vi "Read configuration.vi"(7 "force loading?":bool=TRUE, 8 "error in (no error)":errorcluster, 11 "AOTF in":refnum<class "AOTF.lvclass">) -> (0 "error out":errorcluster, 3 "AOTF out":refnum<class "AOTF.lvclass">)   [LabVIEW 2012, in "AOTF.lvclass"]
doc: "Reads the XML-based configuration file and populates the configuration cluster accordingly. Configuration file name is <component ID>.xml."
uses:
  AOTF.lvclass
  <vilib>/Distrio/Murmex/Murmex/Murmex.lvclass
  AOTF.lvclass/AOTF.ctl
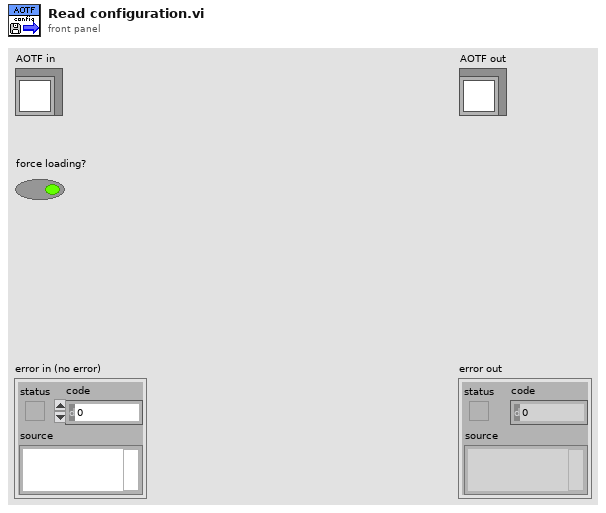
[diagram p1: front panel]
types:
  T1 = typedef "AOTF.lvclass/Configuration cluster.ctl" = cluster{"AO channel":string, "DO lines":string, "LUT path Cluster":cluster{"LUT path Array":path[]}}
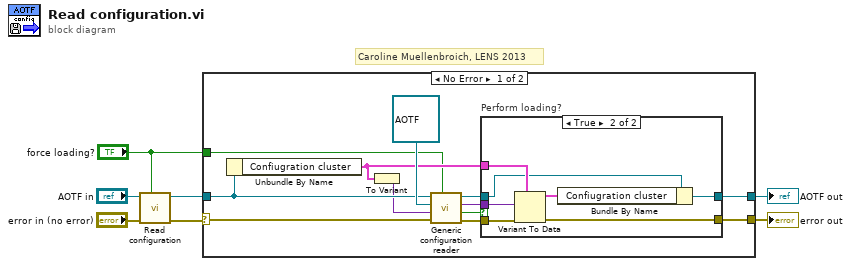
[diagram p0: block diagram]
diagram:
  # "Caroline Muellenbroich, LENS 2013"
  n1 = call-parent "Read configuration.vi"("force loading?"="force loading?", "error in (no error)"="error in (no error)", "Murmex in"="AOTF in") -> ("error out"=w5:errorcluster, "Murmex out"=w4:refnum<class "AOTF.lvclass">)  [unwired: 7 in]
  n2 = case shown="No Error" w5 {
    selector: w5 -> [w16 w30]
    tunnel: w4 -> [w14 w29]
    tunnel: [w18 w30] -> w3
    tunnel: [w19 w29] -> w2
    tunnel: "force loading?" -> [w11 _]
    frame No Error {
      n3 = Unbundle By Name(w14) -> ("Confiugration cluster"=w13:T1)
      n4 = To Variant(anything=w13) -> (Variant=w12:variant)
      n5 = call <vilib>:"Generic configuration reader.vi"("force loading?"=w11, "error in (no error)"=w16, "configuration cluster variant"=w12, "inheritance level"=refnum<class "AOTF.lvclass"> refnum ("AOTF"), "Murmex in"=w14) -> ("error out"=w17:errorcluster, "loaded?"=w8:bool, "configuration data (variant)"=w10:variant, "Murmex out"=w9:refnum<class "AOTF.lvclass">)  [unwired: 3 in]
      n6 = case "Perform loading?" shown="True" w8 {
        tunnel: w13 -> [_ w28]
        tunnel: [w21 w26] -> w18
        tunnel: [w20 w25] -> w19
        tunnel: w17 -> [w21 w22]
        tunnel: w9 -> [w20 w24]
        tunnel: w10 -> [_ w23]
        frame False {
        }
        frame True {
          n7 = Variant To Data(error in=w22, type=w28, Variant=w23) -> (data=w27:T1, error out=w26:errorcluster)
          n8 = Bundle By Name(cluster=w24, "Confiugration cluster"=w27) -> (w25:refnum<class "AOTF.lvclass">)
        }
      }
    }
    frame Error {
    }
  }
  "error out" <- w3
  "AOTF out" <- w2
